vi "reportFAServerStatus.vi"(8 "error in (no error)":errorcluster, 9 "FAIndex":i32, 10 "ModbusBuffer in":refnum<class "ModbusBuffer.lvclass">, 11 "ILCCommunications in":refnum<class "ILCCommunications.lvclass">) -> (0 "error out":errorcluster, 2 "ModbusBuffer out":refnum<class "ModbusBuffer.lvclass">, 3 "ILCCommunications out":refnum<class "ILCCommunications.lvclass">)   [LabVIEW 2016, in "ILCCommunications.lvclass"]
uses:
  ILCCommunications.lvclass
  Common_RT_Modbus/ModbusBuffer/ModbusBuffer.lvclass
  ILCCommunications.lvclass/ILCCommunications.ctl
  Common_RT_ILC/ILC/ILC.lvclass/ILC.ctl
  Common_RT_Modbus/ModbusBuffer/ModbusBuffer.lvclass/ModbusBuffer.ctl
  Common_RT_ILC/ILC/addReportServerStatusFrame.vi
  Common_RT_Modbus/ModbusBuffer/writeHeader.vi
  Common_RT_Modbus/ModbusBuffer/writeU8.vi
  Common_RT_Modbus/ModbusBuffer/writeCRC.vi
  Common_RT_Modbus/ModbusBuffer/writeEndOfFrame.vi
  Common_RT_Modbus/ModbusBuffer/writeWaitForRx.vi
  Common_RT_Modbus/ModbusBuffer/writeByteInstruction.vi
  Common_RT_Modbus/ModbusBuffer/calculateCRC.vi
  Common_RT_FAILC/FAILC/FAILC.lvclass
  D:/Code/ts_M1M3Support/Common_RT_ILC/ILC/ILC.lvclass
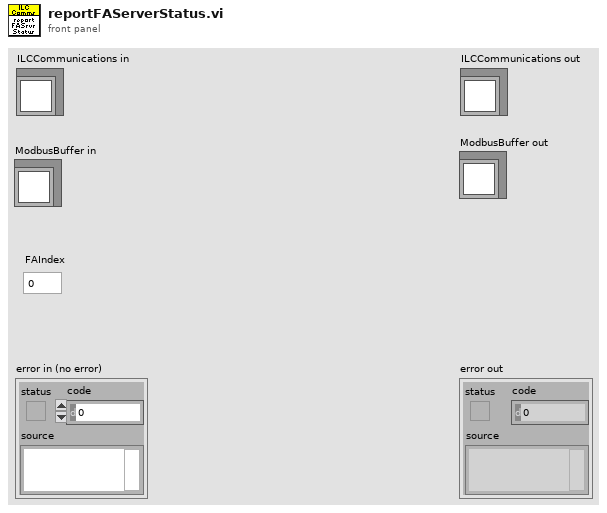
[diagram p1: front panel]
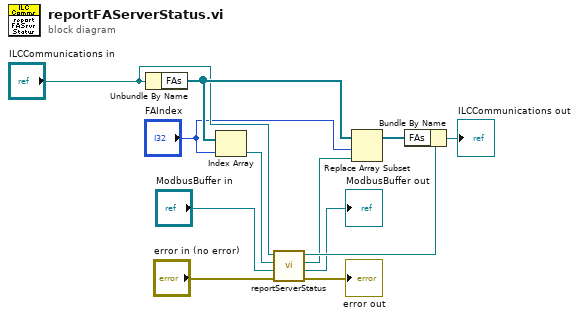
[diagram p0: block diagram]
diagram:
  n1 = Unbundle By Name("ILCCommunications in") -> ("FAs"=w12:refnum<class "FAILC.lvclass">[])
  n2 = Index Array(array=w12, index="FAIndex") -> (element=w4:refnum<class "FAILC.lvclass">)
  n3 = call "reportServerStatus.vi"("error in (no error)"="error in (no error)", "ModbusBuffer in"="ModbusBuffer in", "ILC in"=w4, "ILCCommunications in"="ILCCommunications in") -> ("error out"=→"error out":errorcluster, "ModbusBuffer out"=→"ModbusBuffer out":refnum<class "ModbusBuffer.lvclass">, "ILC out"=w5:refnum<class "FAILC.lvclass">, "ILCCommunications out"=w7:refnum<class "ILCCommunications.lvclass">)  [unwired: 4 in]
  n4 = Replace Array Subset(array=w12, new element=w5, index="FAIndex") -> (w11:refnum<class "FAILC.lvclass">[])
  n5 = Bundle By Name(cluster=w7, "FAs"=w11) -> (→"ILCCommunications out":refnum<class "ILCCommunications.lvclass">)
